vi "ColorSensor.vi"() -> ()   [LabVIEW 2010]
uses:
  <vilib>/NXT/Dual Mode Library/Sensors/Color_Red.vi
  <vilib>/NXT/Dual Mode Library/Sensors/Color_Blue.vi
panel:
  out "Waveform Chart":cluster{"Blue":i16, "Red":i16}(graph)
  out "Red":i16
  out "Blue":i16
  in  "wait":u32=500
  out "Color":string
  in  "stop":bool
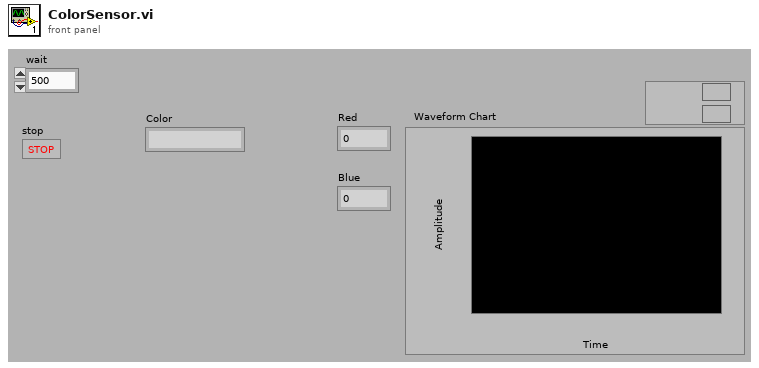
[diagram p1: front panel]
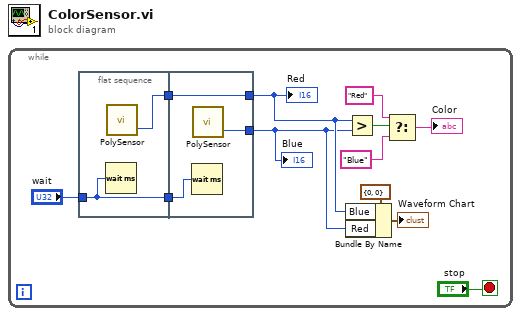
[diagram p0: block diagram]
diagram:
  n1 = while {
    stop <- "stop" stop-if-true
    n2 = flat-sequence {
      tunnel: [w14] -> w11
      tunnel: "wait" -> [w13]
      tunnel: [w13] -> w1
      tunnel: [w17] -> w4
      tunnel: w11 -> [w16]
      tunnel: [w16] -> w5
      tunnel: w1 -> [w15]
      frame #0 {
        n3 = Wait (ms)(milliseconds to wait=w13) -> ()  [unwired: 1 out]
        n4 = call-poly <vilib>:"PolySensor.vi"() -> ("Intensity"=w14:i16)  [unwired: 3 in, 1 out]
      }
      frame #1 {
        n5 = Wait (ms)(milliseconds to wait=w15) -> ()  [unwired: 1 out]
        n6 = call-poly <vilib>:"PolySensor.vi"() -> ("Intensity"=w17:i16)  [unwired: 3 in, 1 out]
      }
    }
    n7 = Bundle By Name(cluster=cluster{"Blue":i16, "Red":i16} {"Blue"=0, "Red"=0} ("input cluster"), "Blue"=w5, "Red"=w4) -> (→"Waveform Chart":cluster{"Blue":i16, "Red":i16})
    n8 = Greater?(x=w5, y=w4) -> (0:w10:bool)
    n9 = Select(t="Red", s=w10, f="Blue") -> (s? t:f=→"Color":string)
    "Blue" <- w4
    "Red" <- w5
  }
